vi "configuration UI.vi"() -> ()   [LabVIEW 2013, in "tag bus configurable plugin editor node.lvclass"]
uses:
  tag bus configurable plugin editor node.lvclass
  <vilib>/NI/Configuration Framework/Node/NodeRef.ctl
  <vilib>/NI/Configuration Framework/Node/NISE_CEF_Node.lvclass
  <vilib>/NI/AMC/Message Queue.ctl
  <vilib>/NI/AMC/Message.ctl
  <vilib>/NI/Tools/Keyed Array/KeyedArray.ctl
  <vilib>/NI/Configuration Framework/Node/UserEventRef.ctl
  <vilib>/NI/Configuration Framework/Controls/EventCluster.ctl
  <vilib>/NI/Configuration Framework/Node/StopEvent.ctl
  <vilib>/NI/Configuration Framework/Node/RefreshUIEvent.ctl
  <vilib>/NI/Configuration Framework/Node/CacheState.ctl
  <vilib>/NI/Configuration Framework/Node/NodeChangeEvent.ctl
  tag bus configurable plugin editor node.lvclass/tag bus configurable plugin editor node.ctl
  <vilib>/NI/Tag Bus/tag/tag descriptor.lvclass/tag descriptor.ctl
  <vilib>/NI/Configuration Framework/serializable configuration/NISE_CEF_serializable configuration.lvclass/NISE_CEF_serializable configuration.ctl
  <vilib>/NI/Tag Bus/tag/write tag name.vi
  <vilib>/Utility/LVClass/Get LV Class Name.vi
  <vilib>/NI/Configuration Framework/error generator.vi
  module/configuration/tag bus configurable plugin module configuration.lvclass
  <vilib>/NI/Module Execution Interface/Engine Configuration/engine configuration.lvclass
  <vilib>/NI/Tag Bus Data Framework/Configuration Editor/Classes/Module editor node/module editor node.lvclass
  <vilib>/NI/Tag Bus Data Framework/Configuration Editor/Classes/Engine Parent/Engine Parent Editor Node.lvclass
  <vilib>/NI/Configuration Framework/serializable configuration/NISE_CEF_serializable configuration.lvclass
  <vilib>/NI/Tag Bus Module Framework/channel/TBM channel.lvclass
  <vilib>/NI/Tools/Keyed Array/Tools_KeyedArray.lvlib
  <vilib>/NI/AMC/AMC.lvlib
  <vilib>/NI/Configuration Framework/NISE_CEF_TreeControl.lvlib
panel:
  in  "node change":T1
  in  "cache state":T2
  in  "refresh UI":T3
  in  "stop event":T4
  in  "Tab Control":enum32{"Static Configuration"}(tab)
  in  "hidden_remove":bool
  in  "hidden_settings":bool
  in  "hidden_Add":bool
  in  "Remove Button":bool
  in  "Add Button":bool
  in  "channel":i32(listbox)
  in  "settings":bool
  in  "user event":T5
  in  "main queue":T6
  in  "node ref":T7
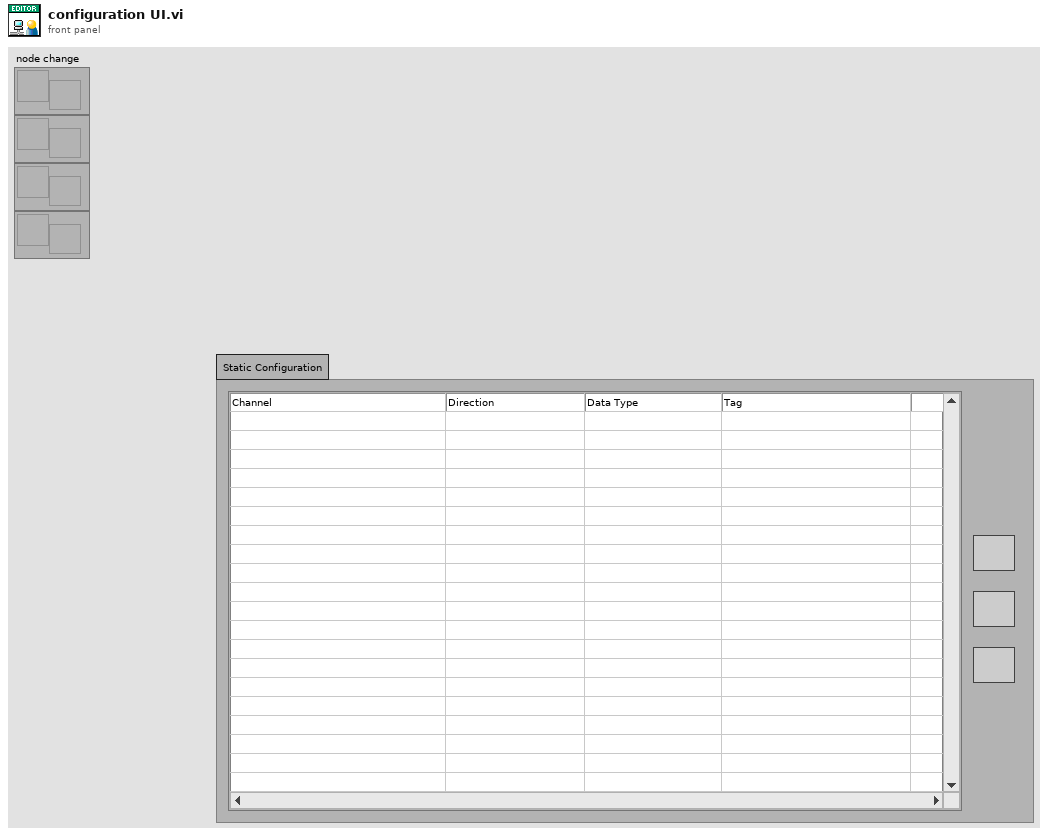
[diagram p1: front panel]
types:
  T1 = typedef "NISE_CEF_Node.lvclass/NodeChangeEvent.ctl" = refnum<user-event>
  T2 = typedef "NISE_CEF_Node.lvclass/CacheState.ctl" = refnum<user-event>
  T3 = typedef "NISE_CEF_Node.lvclass/RefreshUIEvent.ctl" = refnum<user-event>
  T4 = typedef "NISE_CEF_Node.lvclass/StopEvent.ctl" = refnum<user-event>
  T5 = typedef "NISE_CEF_Node.lvclass/UserEventRef.ctl" = refnum<user-event>
  T6 = typedef "AMC.lvlib/Message Queue.ctl" = refnum<queue>
  T7 = typedef "NISE_CEF_Node.lvclass/NodeRef.ctl" = refnum<data-value>
  T8 = typedef "tag bus configurable plugin editor node.lvclass/table line.ctl" = cluster{"channel":refnum<class "TBM channel.lvclass">, "tag name":string}
  T9 = typedef "LVPoint32TypeDef.ctl" = cluster{"Horizontal":i32, "Vertical":i32}
  T10 = typedef "LVRowAndColumnTypeDef.ctl" = cluster{"Row":i32, "Column":i32}
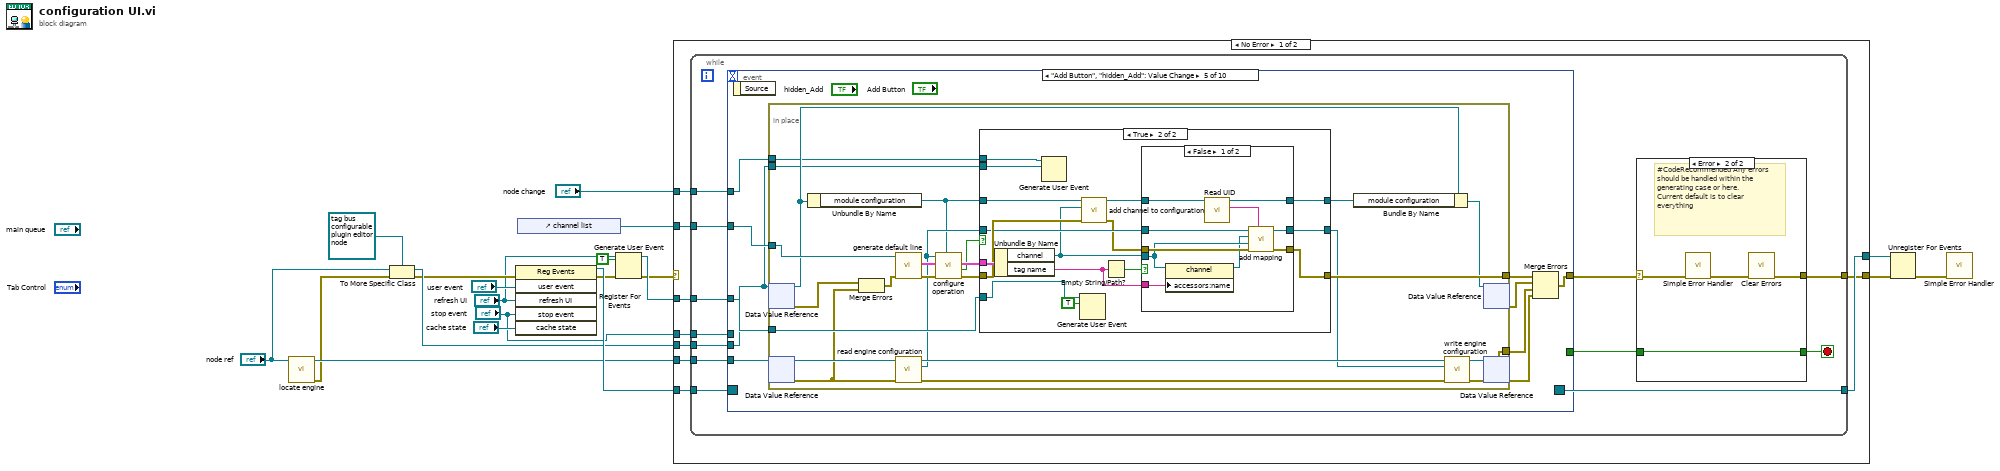
[diagram p0: block diagram]
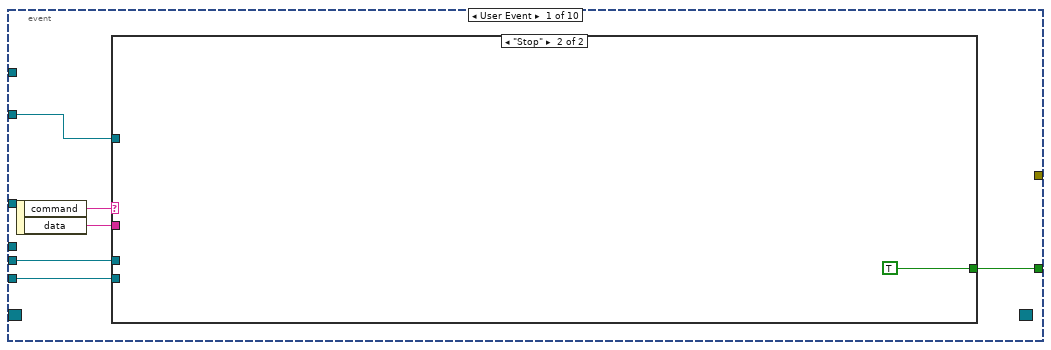
[diagram p3: hidden frame]
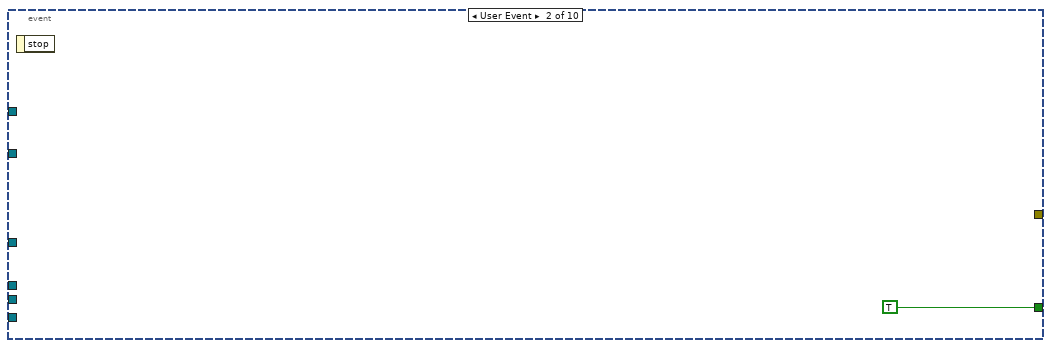
[diagram p5: hidden frame]
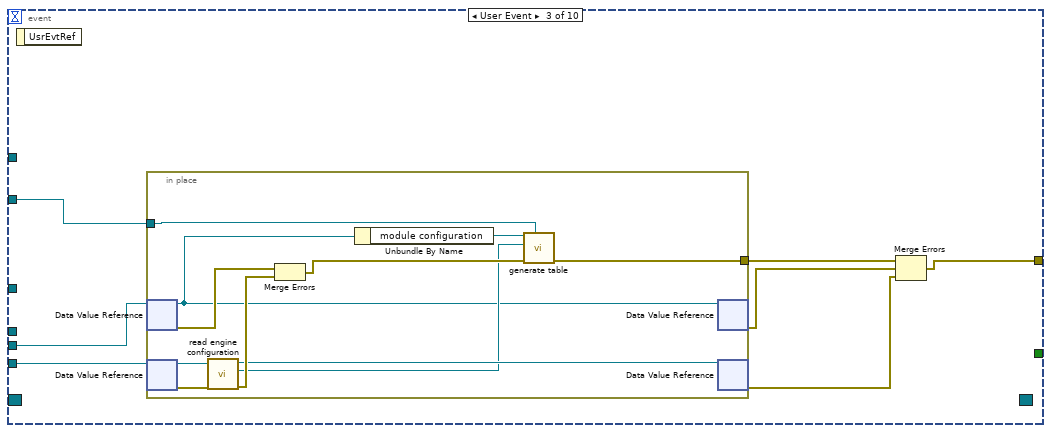
[diagram p6: hidden frame]
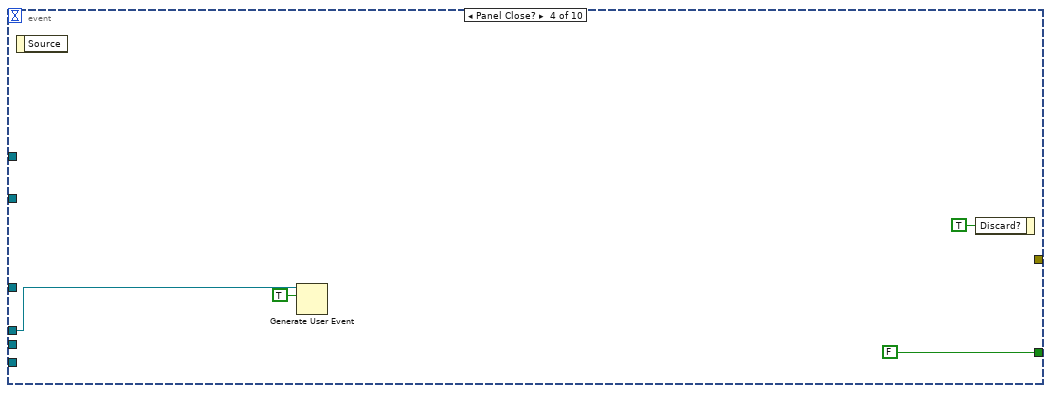
[diagram p7: hidden frame]
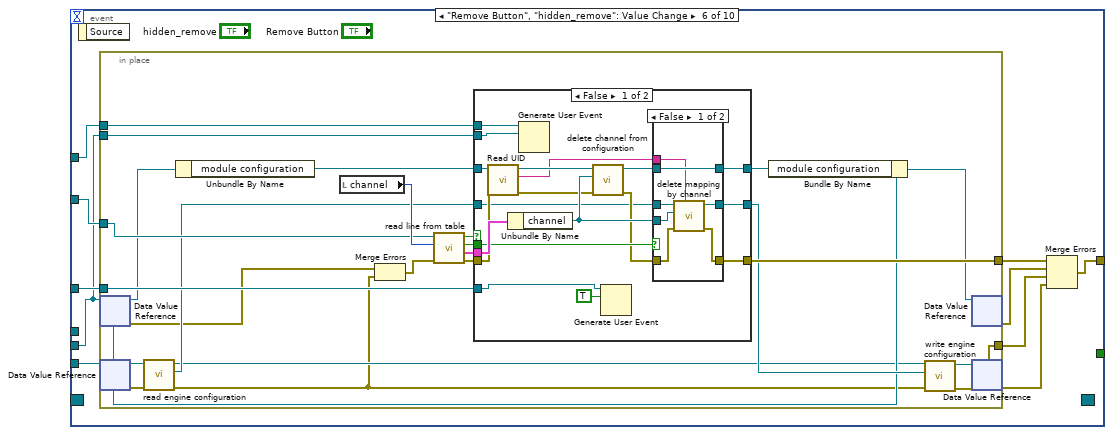
[diagram p10: hidden frame]
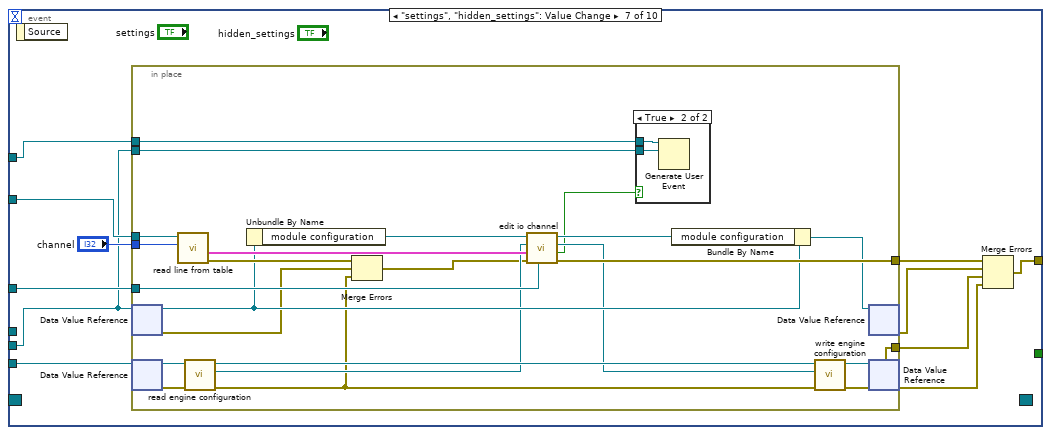
[diagram p13: hidden frame]
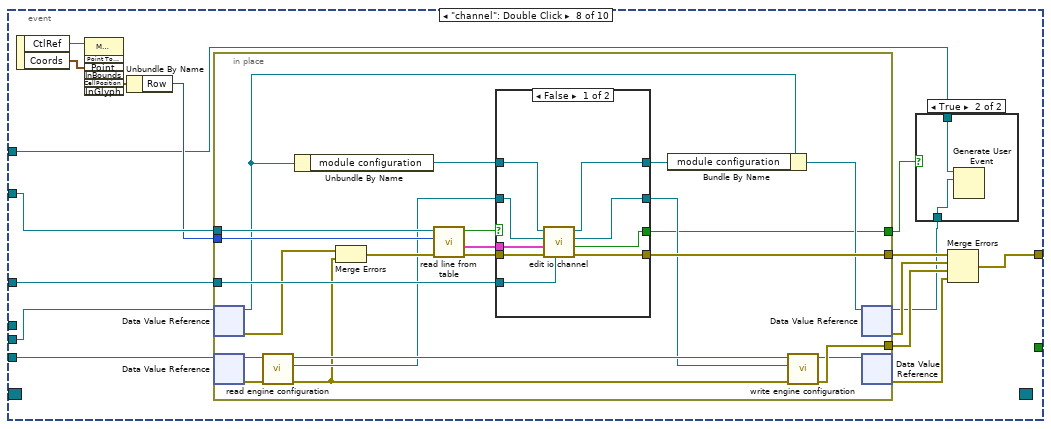
[diagram p15: hidden frame]
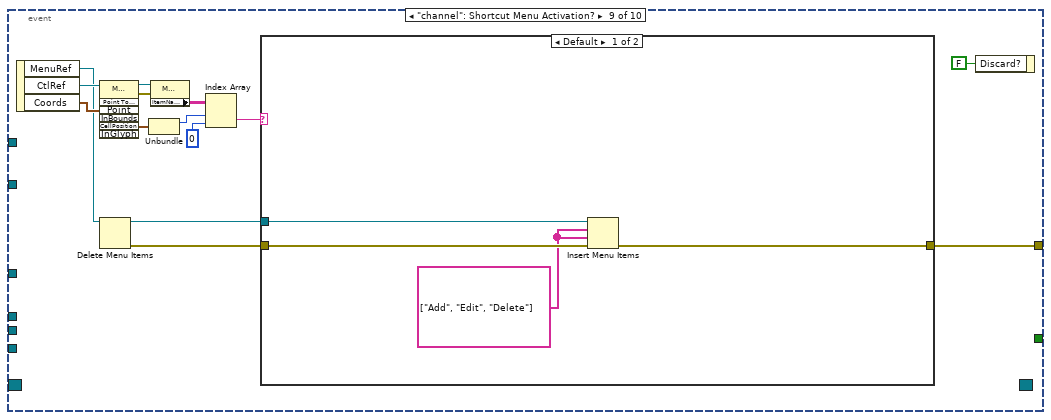
[diagram p18: hidden frame]
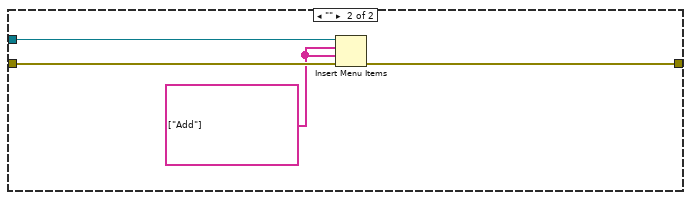
[diagram p19: hidden frame]
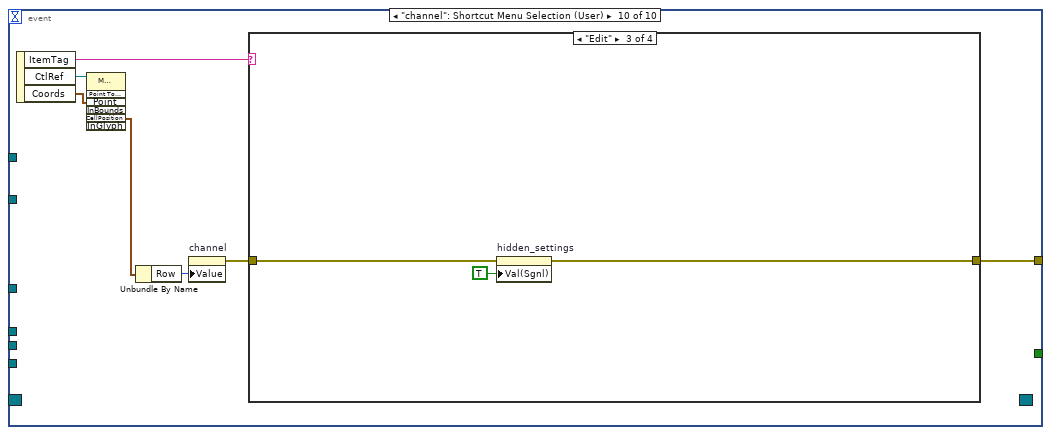
[diagram p20: hidden frame]
diagram:
  n1 = call <vilib>:"locate engine.vi"("component"="node ref") -> ("error out"=w8:errorcluster, "engine"=w15:refnum<data-value>)  [unwired: 9 in]
  n2 = To More Specific Class(target class=refnum<data-value> refnum ("data value reference"), reference="node ref", error in=w8) -> (specific class reference=w11:refnum<data-value>, error out=w10:errorcluster)
  n3 = register-events(error in=w10, "user event", "refresh UI", "stop event", "cache state") -> (reference out=w20:refnum<event-registration>, error out=w16:errorcluster)  [unwired: 1 in]
  n4 = control-ref of="channel list"() -> (w13:refnum<vi>)
  n5 = Generate User Event(user event="refresh UI", event data cluster=TRUE ("event data"), error in=w16) -> (user event out=w7:T3, error out=w2:errorcluster)  [unwired: 1 in]
  n6 = case shown="No Error" w2 {
    selector: w2 -> [_ w337]
    tunnel: w20 -> [w29 w336]
    tunnel: [w28 w336] -> w19
    tunnel: [w27 w337] -> w18
    tunnel: w15 -> [w26 _]
    tunnel: w13 -> [w25 _]
    tunnel: w11 -> [w24 _]
    tunnel: w7 -> [w23 _]
    tunnel: "node change" -> [w22 _]
    tunnel: "stop event" -> [w21 _]
    frame No Error {
      n7 = while {
        tunnel: w29 -> [w41]
        tunnel: [w40] -> w28
        tunnel: w24 -> [w36]
        tunnel: w26 -> [w35]
        tunnel: w23 -> [w34]
        tunnel: w25 -> [w32]
        tunnel: w22 -> [w31]
        tunnel: [w37] -> w27
        tunnel: w21 -> [w30]
        stop <- w39 stop-if-true
        n8 = event shown="[4] \"Add Button\", \"hidden_Add\": Value Change" {
          selector: w41 -> [_ _ _ _ _ _ _ _ _ _]
          dyn-events: [_ _ _ _ _ _ _ _ _ _] -> w40
          timeout: _ -> [_ _ _ _ _ _ _ _ _ _]
          tunnel: [w53 TRUE _ FALSE _ _ _ _ _ _] -> w38
          tunnel: [_ _ w60 _ w84 w149 w215 w253 w297 w322] -> w33
          tunnel: w36 -> [w51 _ w62 _ w79 w144 w210 w249 _ _]
          tunnel: w35 -> [w50 _ w61 _ w83 w150 w214 w250 _ _]
          tunnel: w34 -> [_ _ _ _ w86 w152 w217 w259 _ _]
          tunnel: w32 -> [w48 _ w59 _ w85 w151 w216 w258 _ _]
          tunnel: w31 -> [_ _ _ _ w78 w145 w209 w245 _ _]
          tunnel: w30 -> [_ _ _ w75 _ _ _ _ _ _]
          event User Event {
            n9 = event-data() -> ("command"=w52:string, "data"=w49:string)  [unwired: 1 in]
            n10 = case shown="\"Stop\"" w52 {
              tunnel: [_ TRUE] -> w53
              tunnel: w51 -> [_ _]
              tunnel: w50 -> [_ _]
              tunnel: w49 -> [_ _]
              tunnel: w48 -> [_ _]
              frame Default {
              }
              frame "Stop" {
              }
            }
          }
          event User Event {
            n11 = event-data() -> ()  [unwired: 1 in, 1 out]
          }
          event User Event {
            n12 = event-data() -> ()  [unwired: 1 in, 1 out]
            n13 = in-place {
              in-place-border: [w73] -> w58
              in-place-border: w59 -> [w72]
              n14 = in-place-dvr #1(w62) -> (w64:refnum<class "tag bus configurable plugin editor node.lvclass">, w70:errorcluster)
              n15 = in-place-dvr #2(w61) -> (w67:refnum<class "Engine Parent Editor Node.lvclass">, w69:errorcluster)
              n16 = call <vilib>:"read engine configuration.vi"("error in"=w69, "Engine Parent Editor Node in"=w67) -> ("error out"=w68:errorcluster, "engine configuration"=w65:refnum<class "engine configuration.lvclass">, "Engine Parent Editor Node out"=w66:refnum<class "Engine Parent Editor Node.lvclass">)  [unwired: 7 in]
              n17 = Merge Errors(w70, w68) -> (w71:errorcluster)
              n18 = Unbundle By Name(w64) -> ("module configuration"=w63:refnum<class "tag bus configurable plugin module configuration.lvclass">)
              n19 = call "generate table.vi"("table"=w72, "error in"=w71, "engine configuration"=w65, "tag bus configurable plugin module configuration"=w63) -> ("error out"=w73:errorcluster)  [unwired: 7 in]
              n20 = in-place-dvr #1(w64) -> (w57:errorcluster)  [unwired: 1 out]
              n21 = in-place-dvr #2(w66) -> (w56:errorcluster)  [unwired: 1 out]
            }
            n22 = Merge Errors(w58, w57, w56) -> (w60:errorcluster)
          }
          event Panel Close? {
            n23 = event-data() -> ()  [unwired: 1 in, 1 out]
            n24 = Generate User Event(user event=w75, event data cluster=TRUE ("event data")) -> ()  [unwired: 2 in, 2 out]
            n25 = event-data("Discard?"=TRUE) -> ()  [unwired: 1 in, 1 out]
          }
          event "Add Button", "hidden_Add": Value Change {
            n26 = event-data() -> ()  [unwired: 1 in, 1 out]
            n27 = in-place {
              in-place-border: [w111] -> w87
              in-place-border: w86 -> [w105]
              in-place-border: w85 -> [w104]
              in-place-border: [w99] -> w81
              in-place-border: w79 -> [w89]
              in-place-border: w78 -> [w88]
              n28 = in-place-dvr #3(w79) -> (w92:refnum<class "tag bus configurable plugin editor node.lvclass">, w93:errorcluster)
              n29 = in-place-dvr #4(w83) -> (w102:refnum<class "Engine Parent Editor Node.lvclass">, w101:errorcluster)
              n30 = Unbundle By Name(w92) -> ("module configuration"=w94:refnum<class "tag bus configurable plugin module configuration.lvclass">)
              n31 = Merge Errors(w93, w101) -> (w103:errorcluster)
              n32 = call "generate default line.vi"("error in"=w103, "operations table"=w104) -> ("error out"=w109:errorcluster, "line"=w110:T8)  [unwired: 8 in]
              n33 = call <vilib>:"read engine configuration.vi"("error in"=w101, "Engine Parent Editor Node in"=w102) -> ("error out"=w97:errorcluster, "engine configuration"=w95:refnum<class "engine configuration.lvclass">, "Engine Parent Editor Node out"=w98:refnum<class "Engine Parent Editor Node.lvclass">)  [unwired: 7 in]
              n34 = call "configure operation.vi"("tag bus configurable plugin module configuration"=w94, "error in"=w109, "line item in"=w110, "engine configuration"=w95) -> ("error out"=w107:errorcluster, "success"=w106:bool, "line item out"=w108:T8)  [unwired: 4 in, 1 out]
              n35 = case shown="True" w106 {
                tunnel: [w114 w119] -> w111
                tunnel: w107 -> [w114 w128]
                tunnel: w95 -> [w113 w126]
                tunnel: w108 -> [_ w129]
                tunnel: w94 -> [w112 w130]
                tunnel: [w113 w125] -> w96
                tunnel: [w112 w120] -> w91
                tunnel: w105 -> [_ w118]
                tunnel: w89 -> [_ w116]
                tunnel: w88 -> [_ w115]
                frame False {
                }
                frame True {
                  n36 = Unbundle By Name(w129) -> ("channel"=w123:refnum<class "TBM channel.lvclass">, "tag name"=w122:string)
                  n37 = Generate User Event(user event=w115, event data cluster=w116) -> ()  [unwired: 2 in, 2 out]
                  n38 = Generate User Event(user event=w118, event data cluster=TRUE ("event data")) -> ()  [unwired: 2 in, 2 out]
                  n39 = call "add channel to configuration.vi"("error in"=w128, "channel"=w123, "tag bus configurable plugin module configuration in"=w130) -> ("error out"=w124:errorcluster, "tag bus configurable plugin module configuration out"=w121:refnum<class "tag bus configurable plugin module configuration.lvclass">)  [unwired: 7 in]
                  n40 = Empty String/Path?(string/path=w122) -> (empty?=w127:bool)
                  n41 = case shown="False" w127 {
                    tunnel: w126 -> [w140 w143]
                    tunnel: [w139 w143] -> w125
                    tunnel: w124 -> [w138 w142]
                    tunnel: w123 -> [w137 _]
                    tunnel: w122 -> [w136 _]
                    tunnel: [w134 w142] -> w119
                    tunnel: w121 -> [w133 w141]
                    tunnel: [w132 w141] -> w120
                    frame False {
                      n42 = property class="channel"(reference=w137, "accessors:name"=w136) -> (reference out=w135:refnum<class "TBM channel.lvclass">)  [unwired: 1 in, 1 out]
                      n43 = call <vilib>:"Read UID.vi"("configuration in"=w133) -> ("instance id"=w131:string, "configuration out"=w132:refnum<class "tag bus configurable plugin module configuration.lvclass">)  [unwired: 8 in, 1 out]
                      n44 = call <vilib>:"add mapping.vi"("owner ID"=w131, "error in"=w138, "channel"=w137, "tag descriptor"=w135, "engine configuration"=w140) -> ("error out"=w134:errorcluster, "engine configuration out"=w139:refnum<class "engine configuration.lvclass">)  [unwired: 5 in]
                    }
                    frame True {
                    }
                  }
                }
              }
              n45 = Bundle By Name(cluster=w92, "module configuration"=w91) -> (w90:refnum<class "tag bus configurable plugin editor node.lvclass">)
              n46 = call <vilib>:"write engine configuration.vi"("error in"=w97, "engine configuration"=w96, "Engine Parent Editor Node in"=w98) -> ("error out"=w99:errorcluster, "Engine Parent Editor Node out"=w100:refnum<class "Engine Parent Editor Node.lvclass">)  [unwired: 7 in]
              n47 = in-place-dvr #3(w90) -> (w80:errorcluster)  [unwired: 1 out]
              n48 = in-place-dvr #4(w100) -> (w82:errorcluster)  [unwired: 1 out]
            }
            n49 = Merge Errors(w87, w80, w81, w82) -> (w84:errorcluster)
          }
          event "Remove Button", "hidden_remove": Value Change {
            n50 = event-data() -> ()  [unwired: 1 in, 1 out]
            n51 = in-place {
              in-place-border: [w177] -> w153
              in-place-border: w152 -> [w171]
              in-place-border: w151 -> [w170]
              in-place-border: [w168] -> w146
              in-place-border: w145 -> [w155]
              in-place-border: w144 -> [w154]
              n52 = in-place-dvr #5(w144) -> (w161:refnum<class "tag bus configurable plugin editor node.lvclass">, w156:errorcluster)
              n53 = in-place-dvr #6(w150) -> (w164:refnum<class "Engine Parent Editor Node.lvclass">, w163:errorcluster)
              n54 = call <vilib>:"read engine configuration.vi"("error in"=w163, "Engine Parent Editor Node in"=w164) -> ("error out"=w157:errorcluster, "engine configuration"=w159:refnum<class "engine configuration.lvclass">, "Engine Parent Editor Node out"=w158:refnum<class "Engine Parent Editor Node.lvclass">)  [unwired: 7 in]
              n55 = Unbundle By Name(w161) -> ("module configuration"=w160:refnum<class "tag bus configurable plugin module configuration.lvclass">)
              n56 = local read "channel"() -> (w176:i32)
              n57 = Merge Errors(w156, w157) -> (w162:errorcluster)
              n58 = call "read line from table.vi"("error in"=w162, "line number"=w176, "channels table"=w170) -> ("error out"=w172:errorcluster, "line"=w175:T8, "empty tag?"=w173:bool, "empty channel?"=w174:bool)  [unwired: 5 in]
              n59 = case shown="False" w174 {
                tunnel: [w186 w207] -> w177
                tunnel: w175 -> [w195 _]
                tunnel: w160 -> [w183 w206]
                tunnel: w159 -> [w189 w208]
                tunnel: w173 -> [w194 _]
                tunnel: w172 -> [w192 w207]
                tunnel: [w188 w208] -> w165
                tunnel: [w187 w206] -> w166
                tunnel: w171 -> [w185 _]
                tunnel: w155 -> [w180 _]
                tunnel: w154 -> [w179 _]
                frame False {
                  n60 = call <vilib>:"Read UID.vi"("error in"=w192, "configuration in"=w183) -> ("error out"=w184:errorcluster, "instance id"=w181:string, "configuration out"=w182:refnum<class "tag bus configurable plugin module configuration.lvclass">)  [unwired: 7 in]
                  n61 = Unbundle By Name(w195) -> ("channel"=w193:refnum<class "TBM channel.lvclass">)
                  n62 = Generate User Event(user event=w180, event data cluster=w179) -> ()  [unwired: 2 in, 2 out]
                  n63 = call "delete channel from configuration.vi"("error in"=w184, "channel"=w193, "tag bus configurable plugin module configuration in"=w182) -> ("error out"=w190:errorcluster, "tag bus configurable plugin module configuration out"=w191:refnum<class "tag bus configurable plugin module configuration.lvclass">)  [unwired: 7 in]
                  n64 = Generate User Event(user event=w185, event data cluster=TRUE ("event data")) -> ()  [unwired: 2 in, 2 out]
                  n65 = case shown="False" w194 {
                    tunnel: w193 -> [w201 _]
                    tunnel: w191 -> [w197 w203]
                    tunnel: w190 -> [w200 w204]
                    tunnel: w189 -> [w202 w205]
                    tunnel: [w199 w205] -> w188
                    tunnel: [w198 w204] -> w186
                    tunnel: [w197 w203] -> w187
                    tunnel: w181 -> [w196 _]
                    frame False {
                      n66 = call <vilib>:"delete mapping by channel.vi"("owner ID"=w196, "error in"=w200, "channel"=w201, "engine configuration in"=w202) -> ("error out"=w198:errorcluster, "engine configuration out"=w199:refnum<class "engine configuration.lvclass">)  [unwired: 6 in]
                    }
                    frame True {
                    }
                  }
                }
                frame True {
                }
              }
              n67 = Bundle By Name(cluster=w161, "module configuration"=w166) -> (w167:refnum<class "tag bus configurable plugin editor node.lvclass">)
              n68 = call <vilib>:"write engine configuration.vi"("error in"=w157, "engine configuration"=w165, "Engine Parent Editor Node in"=w158) -> ("error out"=w168:errorcluster, "Engine Parent Editor Node out"=w169:refnum<class "Engine Parent Editor Node.lvclass">)  [unwired: 7 in]
              n69 = in-place-dvr #5(w167) -> (w147:errorcluster)  [unwired: 1 out]
              n70 = in-place-dvr #6(w169) -> (w148:errorcluster)  [unwired: 1 out]
            }
            n71 = Merge Errors(w153, w147, w146, w148) -> (w149:errorcluster)
          }
          event "settings", "hidden_settings": Value Change {
            n72 = event-data() -> ()  [unwired: 1 in, 1 out]
            n73 = in-place {
              in-place-border: [w242] -> w219
              in-place-border: "channel" -> [w239]
              in-place-border: w217 -> [w238]
              in-place-border: w216 -> [w237]
              in-place-border: [w230] -> w211
              in-place-border: w210 -> [w221]
              in-place-border: w209 -> [w220]
              n74 = in-place-dvr #7(w210) -> (w236:refnum<class "tag bus configurable plugin editor node.lvclass">, w223:errorcluster)
              n75 = in-place-dvr #8(w214) -> (w233:refnum<class "Engine Parent Editor Node.lvclass">, w232:errorcluster)
              n76 = call "read line from table.vi"("line number"=w239, "channels table"=w237) -> ("error out"=w241:errorcluster, "line"=w240:T8)  [unwired: 6 in, 2 out]
              n77 = call <vilib>:"read engine configuration.vi"("error in"=w232, "Engine Parent Editor Node in"=w233) -> ("error out"=w224:errorcluster, "engine configuration"=w226:refnum<class "engine configuration.lvclass">, "Engine Parent Editor Node out"=w228:refnum<class "Engine Parent Editor Node.lvclass">)  [unwired: 7 in]
              n78 = Unbundle By Name(w236) -> ("module configuration"=w229:refnum<class "tag bus configurable plugin module configuration.lvclass">)
              n79 = Merge Errors(w241, w223, w224) -> (w225:errorcluster)
              n80 = call "edit io channel.vi"("refresh UI"=w238, "error in"=w225, "line"=w240, "engine configuration in"=w226, "tag bus configurable plugin module configuration in"=w229) -> ("error out"=w242:errorcluster, "change?"=w222:bool, "engine configuration"=w227:refnum<class "engine configuration.lvclass">, "tag bus configurable plugin module configuration out"=w234:refnum<class "tag bus configurable plugin module configuration.lvclass">)  [unwired: 3 in]
              n81 = case shown="True" w222 {
                tunnel: w221 -> [_ w244]
                tunnel: w220 -> [_ w243]
                frame False {
                }
                frame True {
                  n82 = Generate User Event(user event=w243, event data cluster=w244) -> ()  [unwired: 2 in, 2 out]
                }
              }
              n83 = Bundle By Name(cluster=w236, "module configuration"=w234) -> (w235:refnum<class "tag bus configurable plugin editor node.lvclass">)
              n84 = call <vilib>:"write engine configuration.vi"("error in"=w224, "engine configuration"=w227, "Engine Parent Editor Node in"=w228) -> ("error out"=w230:errorcluster, "Engine Parent Editor Node out"=w231:refnum<class "Engine Parent Editor Node.lvclass">)  [unwired: 7 in]
              n85 = in-place-dvr #7(w235) -> (w212:errorcluster)  [unwired: 1 out]
              n86 = in-place-dvr #8(w231) -> (w213:errorcluster)  [unwired: 1 out]
            }
            n87 = Merge Errors(w219, w212, w211, w213) -> (w215:errorcluster)
          }
          event "channel": Double Click {
            n88 = event-data() -> ("CtlRef"=w257:refnum<vi>, "Coords"=w256:T9)  [unwired: 1 in]
            n89 = invoke class="MCListbox (strict)" method="Point To Row Column"(reference=w257, "Point"=w256) -> ("CellPosition"=w255:T10)  [unwired: 5 in, 6 out]
            n90 = Unbundle By Name(w255) -> ("Row"=w254:i32)
            n91 = in-place {
              in-place-border: [w284] -> w260
              in-place-border: w259 -> [w281]
              in-place-border: w258 -> [w280]
              in-place-border: w254 -> [w279]
              in-place-border: [w276] -> w248
              in-place-border: [w263] -> w247
              n92 = in-place-dvr #9(w249) -> (w265:refnum<class "tag bus configurable plugin editor node.lvclass">, w270:errorcluster)
              n93 = in-place-dvr #10(w250) -> (w274:refnum<class "Engine Parent Editor Node.lvclass">, w273:errorcluster)
              n94 = call <vilib>:"read engine configuration.vi"("error in"=w273, "Engine Parent Editor Node in"=w274) -> ("error out"=w269:errorcluster, "engine configuration"=w271:refnum<class "engine configuration.lvclass">, "Engine Parent Editor Node out"=w272:refnum<class "Engine Parent Editor Node.lvclass">)  [unwired: 7 in]
              n95 = Unbundle By Name(w265) -> ("module configuration"=w264:refnum<class "tag bus configurable plugin module configuration.lvclass">)
              n96 = Merge Errors(w270, w269) -> (w277:errorcluster)
              n97 = call "read line from table.vi"("error in"=w277, "line number"=w279, "channels table"=w280) -> ("error out"=w283:errorcluster, "line"=w282:T8, "empty channel?"=w278:bool)  [unwired: 5 in, 1 out]
              n98 = case shown="False" w278 {
                tunnel: [w293 w294] -> w284
                tunnel: w283 -> [w292 w294]
                tunnel: w282 -> [w291 _]
                tunnel: w271 -> [w290 w295]
                tunnel: w264 -> [w289 w296]
                tunnel: [w288 w296] -> w267
                tunnel: [w287 w295] -> w268
                tunnel: w281 -> [w286 _]
                tunnel: [w285 _] -> w263
                frame False {
                  n99 = call "edit io channel.vi"("refresh UI"=w286, "error in"=w292, "line"=w291, "engine configuration in"=w290, "tag bus configurable plugin module configuration in"=w289) -> ("error out"=w293:errorcluster, "change?"=w285:bool, "engine configuration"=w287:refnum<class "engine configuration.lvclass">, "tag bus configurable plugin module configuration out"=w288:refnum<class "tag bus configurable plugin module configuration.lvclass">)  [unwired: 3 in]
                }
                frame True {
                }
              }
              n100 = Bundle By Name(cluster=w265, "module configuration"=w267) -> (w266:refnum<class "tag bus configurable plugin editor node.lvclass">)
              n101 = call <vilib>:"write engine configuration.vi"("error in"=w269, "engine configuration"=w268, "Engine Parent Editor Node in"=w272) -> ("error out"=w276:errorcluster, "Engine Parent Editor Node out"=w275:refnum<class "Engine Parent Editor Node.lvclass">)  [unwired: 7 in]
              n102 = in-place-dvr #9(w266) -> (w246:refnum<data-value>, w251:errorcluster)
              n103 = in-place-dvr #10(w275) -> (w252:errorcluster)  [unwired: 1 out]
            }
            n104 = case shown="True" w247 {
              tunnel: w246 -> [_ w262]
              tunnel: w245 -> [_ w261]
              frame False {
              }
              frame True {
                n105 = Generate User Event(user event=w261, event data cluster=w262) -> ()  [unwired: 2 in, 2 out]
              }
            }
            n106 = Merge Errors(w260, w251, w248, w252) -> (w253:errorcluster)
          }
          event "channel": Shortcut Menu Activation? {
            n107 = event-data() -> ("MenuRef"=w307:refnum<k9>, "CtlRef"=w309:refnum<vi>, "Coords"=w308:T9)  [unwired: 1 in]
            n108 = invoke class="MCListbox (strict)" method="Point To Row Column"(reference=w309, "Point"=w308) -> (reference out=w306:refnum<vi>, error out=w305:errorcluster, "CellPosition"=w304:T10)  [unwired: 5 in, 4 out]
            n109 = Delete Menu Items(9:w307) -> (0:w298:errorcluster, 3:w299:refnum<k9>)  [unwired: 3 in]
            n110 = Unbundle(w304) -> ("Row"=w302:i32)  [unwired: 1 out]
            n111 = property class="MCListbox (strict)"(reference=w306, error in=w305) -> ("ItemNames"=w303:string[][])  [unwired: 2 out]
            n112 = Index Array(array=w303, index (row)=w302, index (col)=0 ("disabled index (col)")) -> (element=w300:string)
            n113 = case shown="Default" w300 {
              tunnel: w299 -> [w314 w318]
              tunnel: w298 -> [w313 w317]
              tunnel: [w312 w316] -> w297
              frame Default {
                w311 = string[] ["Add", "Edit", "Delete"] ("item names")
                n114 = Insert Menu Items(6:w313, 7:w311, 8:w311, 9:w314) -> (0:w312:errorcluster)  [unwired: 2 in, 2 out]
              }
              frame "" {
                w315 = string[] ["Add"] ("item names")
                n115 = Insert Menu Items(6:w317, 7:w315, 8:w315, 9:w318) -> (0:w316:errorcluster)  [unwired: 2 in, 2 out]
              }
            }
            n116 = event-data("Discard?"=FALSE) -> ()  [unwired: 1 in, 1 out]
          }
          event "channel": Shortcut Menu Selection (User) {
            n117 = event-data() -> ("ItemTag"=w323:string, "CtlRef"=w324:refnum<vi>, "Coords"=w325:T9)  [unwired: 1 in]
            n118 = invoke class="MCListbox (strict)" method="Point To Row Column"(reference=w324, "Point"=w325) -> ("CellPosition"=w320:T10)  [unwired: 5 in, 6 out]
            n119 = Unbundle By Name(w320) -> ("Row"=w319:i32)
            n120 = property on="channel" class="MCListbox (strict)"("Value"=w319) -> (error out=w321:errorcluster)  [unwired: 2 in, 1 out]
            n121 = case shown="\"Edit\"" w323 {
              tunnel: w321 -> [w326 w328 w332 w335]
              tunnel: [w326 w327 w331 w334] -> w322
              frame Default {
              }
              frame "Add" {
                n122 = property on="hidden_Add" class="Bool (strict)"(error in=w328, "Val(Sgnl)"=TRUE ("Value (Signaling)")) -> (error out=w327:errorcluster)  [unwired: 1 in, 1 out]
              }
              frame "Edit" {
                n123 = property on="hidden_settings" class="Bool (strict)"(error in=w332, "Val(Sgnl)"=TRUE ("Value (Signaling)")) -> (error out=w331:errorcluster)  [unwired: 1 in, 1 out]
              }
              frame "Delete" {
                n124 = property on="hidden_remove" class="Bool (strict)"(error in=w335, "Val(Sgnl)"=FALSE ("Value (Signaling)")) -> (error out=w334:errorcluster)  [unwired: 1 in, 1 out]
              }
            }
          }
        }
        n125 = case shown="Error" w33 {
          selector: w33 -> [w42 w46]
          tunnel: [w43 w47] -> w39
          tunnel: w38 -> [w43 w47]
          tunnel: [w42 w44] -> w37
          frame No Error {
          }
          frame Error {
            # "#CodeRecommended Any errors should be handled within the generating case or here. Current default is to clear everything"
            n126 = call <vilib>:"Simple Error Handler.vi"("error in (no error)"=w46) -> ("error out"=w45:errorcluster)  [unwired: 4 in, 4 out]
            n127 = call <vilib>:"Clear Errors.vi"("error in (no error)"=w45) -> ("error out"=w44:errorcluster)  [unwired: 6 in]
          }
        }
      }
    }
    frame Error {
    }
  }
  n128 = Unregister For Events(event registration refnum=w19, error in=w18) -> (error out=w14:errorcluster)
  n129 = call <vilib>:"Simple Error Handler.vi"("error in (no error)"=w14) -> ()  [unwired: 4 in, 5 out]
